vi "Vacuum Off.vi"() -> (0 "error out":errorcluster)   [LabVIEW 2025]
doc: "Turns off the Vacuum table so that the UUT can be safely removed from the test fixture."
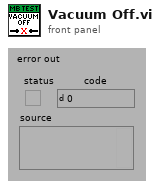
[diagram p1: front panel]
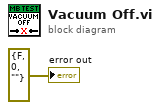
[diagram p0: block diagram]
diagram:
  "error out" <- errorcluster {"status"=FALSE, "code"=0, "source"=""} ("error out")
